vi "Dialogue_OneButton.vi"(6 "Btn_1 Text":string="OK", 8 "error in":errorcluster, 10 "Message":string, 11 "Title":string) -> (0 "error out":errorcluster, 3 "Btn_1?":bool=TRUE)   [LabVIEW 2014, in "hse-ui.lvlib"]
doc: "Shows a dialog window with a message and an OK button\n\n____\nHAMPEL SOFTWARE ENGINEERING v0.7.0 (2018-07-16 18:12)"
uses:
  hse-ui.lvlib
  FPControl/FPControl_Actions.ctl
panel:
  in  "Btn_OK":bool
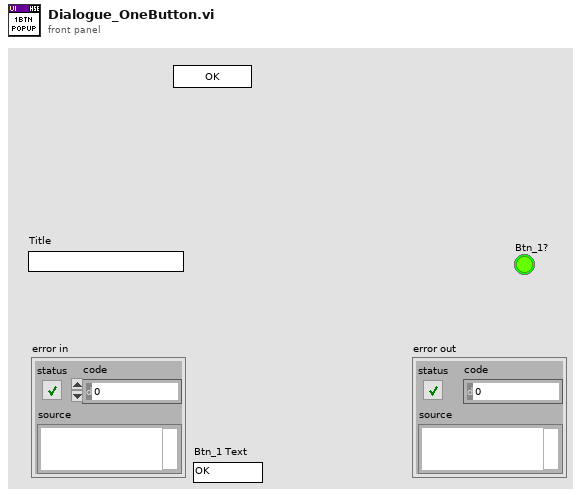
[diagram p1: front panel]
types:
  T1 = typedef "hse-ui.lvlib/FPControl_Actions.ctl" = enum16{"Open", "Hide", "Close", "Bring To Front", "Center", "Minimize", "Maximize"}
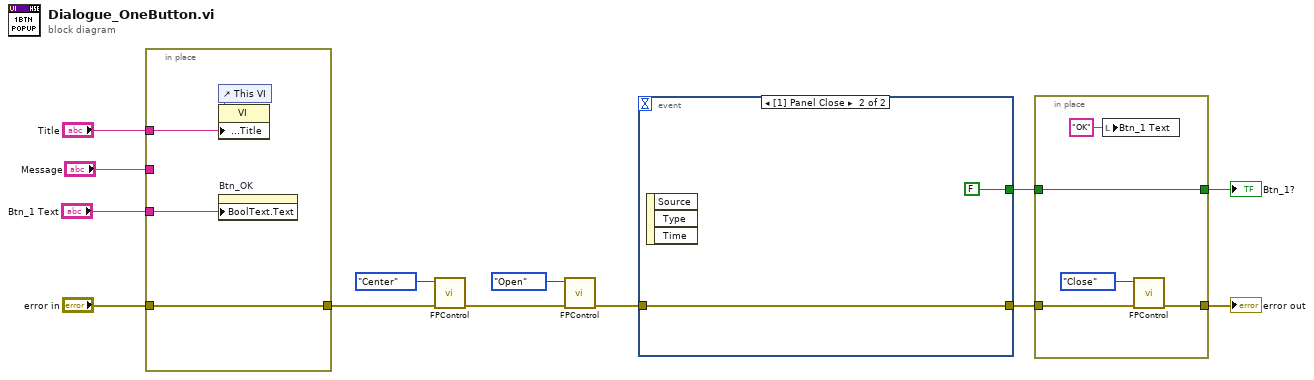
[diagram p0: block diagram]
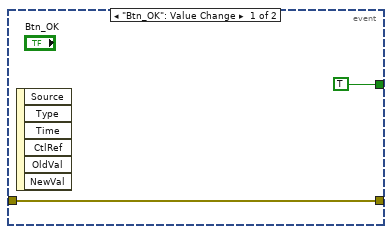
[diagram p2: hidden frame]
diagram:
  n1 = in-place {
    in-place-border: "error in" -> [w17]
    in-place-border: [w17] -> w7
    in-place-border: "Title" -> [w15]
    in-place-border: "Message" -> [_]
    in-place-border: "Btn_1 Text" -> [w14]
    n2 = control-ref of="This VI"() -> (w16:refnum<vi>)
    n3 = property class="VI"(reference=w16, "Front Panel.Title"=w15) -> ()  [unwired: 1 in, 2 out]
    n4 = property on="Btn_OK" class="Bool"("BoolText.Text"=w14) -> ()  [unwired: 2 in, 2 out]
  }
  n5 = call "FPControl.vi"("error in"=w7, "Function"=FPControl_Actions."Center") -> ("error out"=w11:errorcluster)  [unwired: 9 out]
  n6 = call "FPControl.vi"("error in"=w11, "Function"=FPControl_Actions."Open") -> ("error out"=w5:errorcluster)  [unwired: 9 out]
  n7 = event shown="[1] Panel Close" {
    selector: _ -> [_ _]
    dyn-events: _ -> [_ _]
    timeout: _ -> [_ _]
    tunnel: w5 -> [w19 w21]
    tunnel: [w19 w21] -> w9
    tunnel: [TRUE FALSE] -> w2
    event "Btn_OK": Value Change {
      n8 = event-data() -> ()  [unwired: 1 in, 6 out]
    }
    event Panel Close {
      n9 = event-data() -> ()  [unwired: 1 in, 3 out]
    }
  }
  n10 = in-place {
    in-place-border: [w25] -> w10
    in-place-border: w9 -> [w24]
    in-place-border: w2 -> [w22]
    in-place-border: [w22] -> w1
    n11 = local write "Btn_1 Text"("OK" ("Btn_1 Text")) -> ()
    n12 = call "FPControl.vi"("error in"=w24, "Function"=FPControl_Actions."Close") -> ("error out"=w25:errorcluster)  [unwired: 9 out]
  }
  "error out" <- w10
  "Btn_1?" <- w1
